vi "Update Animation.vi"(11 "Deployable in":refnum<class "Zap Sat.lvclass">) -> (3 "Deployable out":refnum<class "Zap Sat.lvclass">)   [LabVIEW 2021, in "Zap Sat.lvclass"]
uses:
  Zap Sat.lvclass
  Zap Sat.lvclass/Zap Sat.ctl
  Math/Math.lvlib
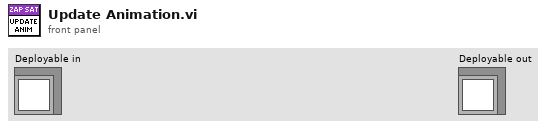
[diagram p1: front panel]
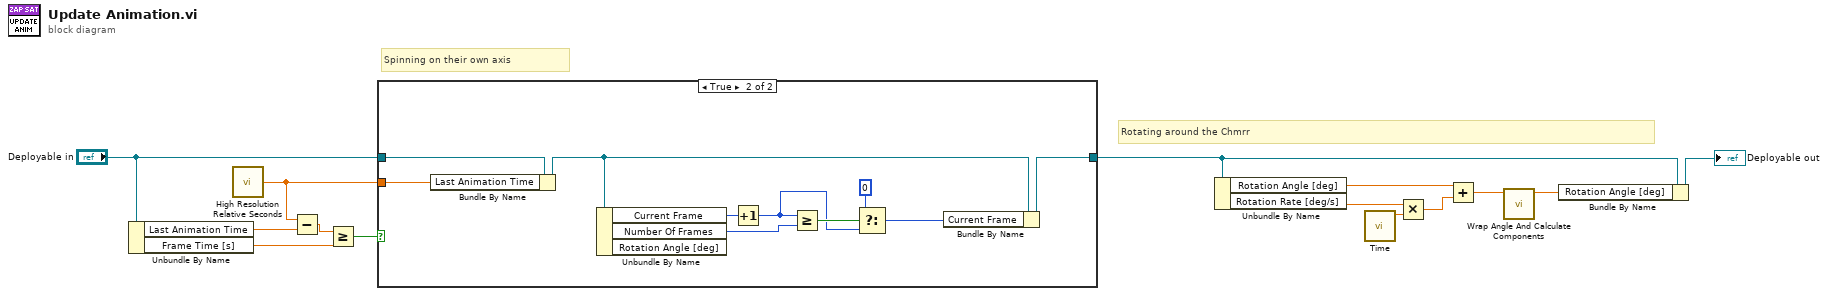
[diagram p0: block diagram]
diagram:
  # "Rotating around the Chmrr"
  # "Spinning on their own axis"
  n1 = Unbundle By Name("Deployable in") -> ("Last Animation Time"=w12:dbl, "Frame Time [s]"=w14:dbl)
  n2 = call <vilib>:"High Resolution Relative Seconds.vi"() -> ("relative seconds"=w9:dbl)
  n3 = Subtract(x=w9, y=w12) -> (x-y=w13:dbl)
  n4 = Greater Or Equal?(x=w13, y=w14) -> (x >= y?=w10:bool)
  n5 = case shown="True" w10 {
    tunnel: [w15 w23] -> w7
    tunnel: "Deployable in" -> [w15 w25]
    tunnel: w9 -> [_ w16]
    frame False {
    }
    frame True {
      n6 = Bundle By Name(cluster=w25, "Last Animation Time"=w16) -> (w24:refnum<class "Zap Sat.lvclass">)
      n7 = Unbundle By Name(w24) -> ("Current Frame"=w21:i32, "Number Of Frames"=w20:i32)  [unwired: 1 out]
      n8 = Increment(x=w21) -> (x+1=w17:i32)
      n9 = Greater Or Equal?(x=w17, y=w20) -> (x >= y?=w19:bool)
      n10 = Select(t=0, s=w19, f=w17) -> (s? t:f=w22:i32)
      n11 = Bundle By Name(cluster=w24, "Current Frame"=w22) -> (w23:refnum<class "Zap Sat.lvclass">)
    }
  }
  n12 = Unbundle By Name(w7) -> ("Rotation Angle [deg]"=w6:sgl, "Rotation Rate [deg/s]"=w3:sgl)
  n13 = call "Time.vi"() -> ("Delta Time [s]"=w2:sgl)  [unwired: 10 in, 1 out]
  n14 = Multiply(x=w3, y=w2) -> (x*y=w1:sgl)
  n15 = Add(x=w6, y=w1) -> (x+y=w5:sgl)
  n16 = call "Wrap Angle And Calculate Components.vi"("Angle in [deg]"=w5) -> ("Angle out [deg]"=w4:sgl)  [unwired: 10 in]
  n17 = Bundle By Name(cluster=w7, "Rotation Angle [deg]"=w4) -> (→"Deployable out":refnum<class "Zap Sat.lvclass">)
